vi "X_Q_2500.vi"(9 "Type":string) -> (0 "Qn":dbl[](array[numeric]), 2 "L":i32)   [LabVIEW 2015]
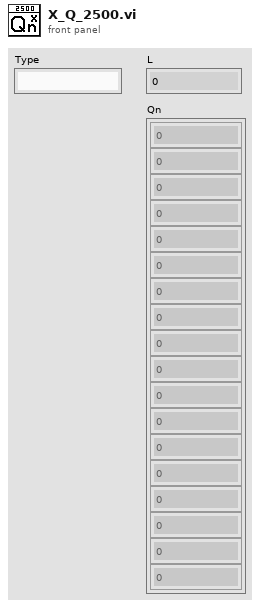
[diagram p1: front panel]
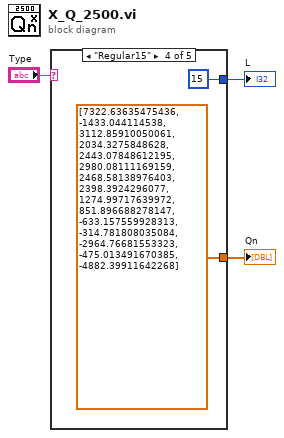
[diagram p0: block diagram]
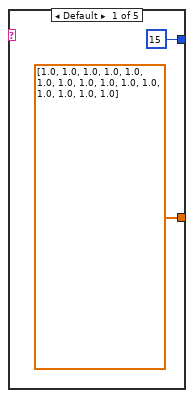
[diagram p2: hidden frame]
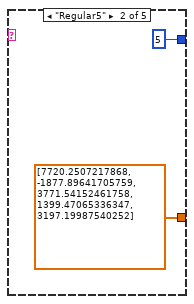
[diagram p3: hidden frame]
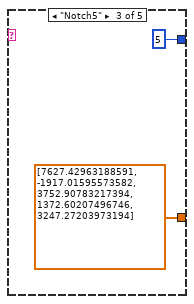
[diagram p4: hidden frame]
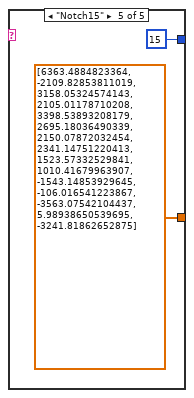
[diagram p5: hidden frame]
diagram:
  n1 = case shown="\"Regular15\"" "Type" {
    tunnel: [15 5 5 15 15] -> w2
    tunnel: [dbl[] [1.0, 1.0, 1.0, 1.0, 1.0, 1.0, 1.0, 1.0, 1.0, 1.0, 1.0, 1.0, 1.0, 1.0, 1.0] ("Qn") dbl[] [7720.2507217868, -1877.89641705759, 3771.54152461758, 1399.47065336347, 3197.19987540252] ("Qn") dbl[] [7627.42963188591, -1917.01595573582, 3752.90783217394, 1372.60207496746, 3247.27203973194] ("Qn") dbl[] [7322.63635475436, -1433.044114538, 3112.85910050061, 2034.3275848628, 2443.07848612195, 2980.08111169159, 2468.58138976403, 2398.3924296077, 1274.99717639972, 851.896688278147, -633.157559928313, -314.781808035084, -2964.76681553323, -475.013491670385, -4882.39911642268] ("Qn") dbl[] [6363.4884823364, -2109.82853811019, 3158.05324574143, 2105.01178710208, 3398.53893208179, 2695.18036490339, 2150.07872032454, 2341.14751220413, 1523.57332529841, 1010.41679963907, -1543.14853929645, -106.016541223867, -3563.07542104437, 5.98938650539695, -3241.81862652875] ("Qn")] -> w1
    frame Default {
    }
    frame "Regular5" {
    }
    frame "Notch5" {
    }
    frame "Regular15" {
    }
    frame "Notch15" {
    }
  }
  "Qn" <- w1
  "L" <- w2
